vi "RemoveTrendPoint.vi"(10 "TrendPoints id":string, 11 "TrendPoints in":T1[](array[typedef])) -> (3 "TrendPoints out":T1[](array[typedef]))   [LabVIEW 2017, in "McsaStartupAnalysis.lvlib"]
uses:
  <vilib>/addons/InsightCM/Devices/Shared/Mcsa/McsaStartupAnalysis/McsaStartupAnalysis.lvlib
  <vilib>/addons/InsightCM/MessageBus/Base/controls/TrendPoint.ctl
  <vilib>/addons/InsightCM/MessageBus/Base/controls/KeyValuePair.ctl
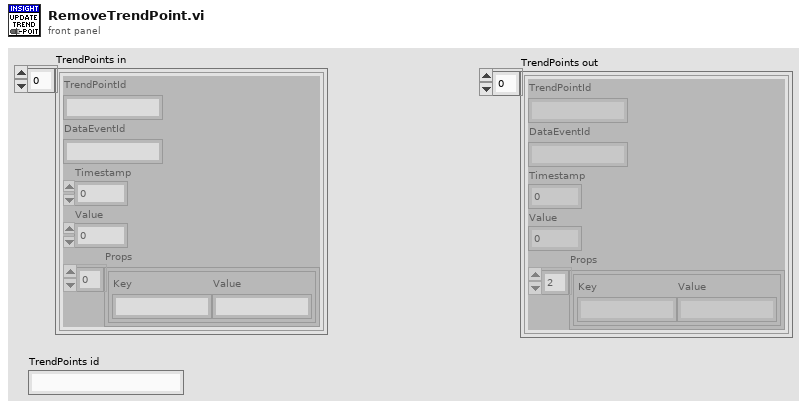
[diagram p1: front panel]
types:
  T1 = typedef "TrendPoint.ctl" = cluster{"TrendPointId":string, "DataEventId":string, "Timestamp":i64, "Value":dbl, "Props":T2[]}
  T2 = typedef "KeyValuePair.ctl" = cluster{"Key":string, "Value":string}
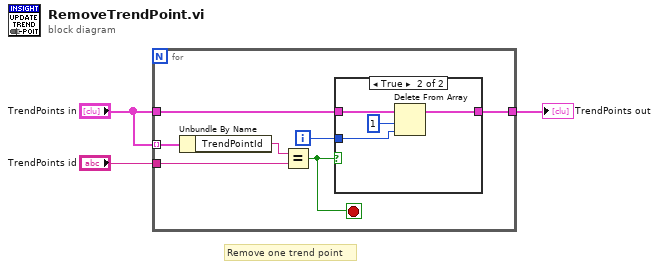
[diagram p0: block diagram]
diagram:
  # "Remove one trend point"
  n1 = for {
    tunnel: "TrendPoints in" -> [w8] mode=indexing
    tunnel: "TrendPoints id" -> [w9]
    tunnel: "TrendPoints in" -> [w7]
    tunnel: [w6] -> w1
    i -> [w5]
    stop <- w4 stop-if-true
    n2 = Unbundle By Name(w8) -> ("TrendPointId"=w10:string)
    n3 = Equal?(x=w10, y=w9) -> (x = y?=w4:bool)
    n4 = case shown="True" w4 {
      tunnel: w7 -> [w11 w15]
      tunnel: [w11 w14] -> w6
      tunnel: w5 -> [_ w12]
      frame False {
      }
      frame True {
        n5 = Delete From Array(array=w15, length=1 ("index"), index=w12) -> (array with subset deleted=w14:T1[])  [unwired: 1 out]
      }
    }
  }
  "TrendPoints out" <- w1
